vi "__SR530_read.vi"(7 "GPIB":string="29") -> (1 "Phase":dbl=-0.002487, 3 "R":dbl=0.0002225)   [LabVIEW 2017]
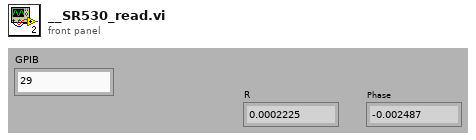
[diagram p1: front panel]
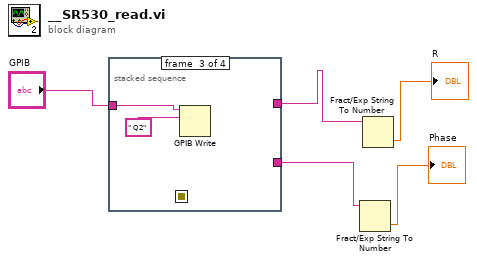
[diagram p0: block diagram]
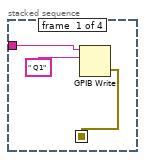
[diagram p2: hidden frame]
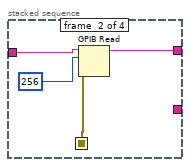
[diagram p3: hidden frame]
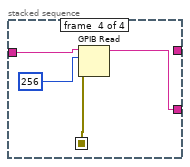
[diagram p4: hidden frame]
diagram:
  n1 = stacked-sequence {
    seq-local: [w6 _ _ _] -> [_ w10 _ w16]
    tunnel: "GPIB" -> [w8 w12 w14 w18]
    tunnel: [_ w9 _ _] -> w4
    tunnel: [_ _ _ w15] -> w1
    frame #0 {
      n2 = GPIB Write(0:w8, 1:" Q1") -> (6:w6:errorcluster)  [unwired: 3 in, 1 out]
    }
    frame #1 {
      n3 = GPIB Read(0:w12, 1:256, 3:w10) -> (5:w9:string)  [unwired: 2 in, 2 out]
    }
    frame #2 {
      n4 = GPIB Write(0:w14, 1:" Q2") -> ()  [unwired: 3 in, 2 out]
    }
    frame #3 {
      n5 = GPIB Read(0:w18, 1:256, 3:w16) -> (5:w15:string)  [unwired: 2 in, 2 out]
    }
  }
  n6 = Fract/Exp String To Number(string=w1) -> (number=→"Phase":dbl)  [unwired: 3 in, 1 out]
  n7 = Fract/Exp String To Number(string=w4) -> (number=→"R":dbl)  [unwired: 3 in, 1 out]
